vi "sql-readinfo_vfixture.vi"(0 "DBSet":T1={"Server"="172.20.23.107", "DB"="HTPSDB", "PSW"="data'songyy", "User"="sa"}, 5 "操作模式":T2(ring)=enum."查询数据", 7 "查询项目":string="LuxsharePN,CustomerPN,Customer,SampleDes,AWG,Length,EEPROMWrite,LabelPrint,Remarks", 11 "标识列":string, 12 "限定条件":string="where LuxsharePN='L12345678'", 13 "Page":string, 15 "Desc":string) -> (14 "数据输出2":dbl[][](array[numeric]), 16 "错误类型":string, 17 "StringArray2":string[][](array[string])=[["L12345678\t\tIBM\t40G Ethernet QSFP+ Passive DAC Cable\t28\t3000\t0\t0\trefer to IBM Spec"]], 18 "列内对数":i32=1, 19 "返回记录数目":i32=1, 20 "ConvertToArray":string[][](array[string])=[["L12345678", "", "IBM", "40G Ethernet QSFP+ Passive DAC Cable", "28", "3000", "0", "0", "refer to IBM Spec"]], 21 "status":bool, 23 "ResultString":string="L12345678\t\tIBM\t40G Ethernet QSFP+ Passive DAC Cable\t28\t3000\t0\t0\trefer to IBM Spec\r", 24 "ConvertToClusterArray":cluster{"项":string, "值":string}[](array[cluster])=[{"项"="", "值"=""}, {"项"="L12345678", "值"="L12345678"}], 25 "DataPair":dbl[](array[numeric]), 27 "数据输出":dbl[][](array[numeric]))   [LabVIEW 2011]
panel:
  out "错误输出 2":errorcluster caption="错误输出"
  out "result string":string="select LuxsharePN,CustomerPN,Customer,SampleDes,AWG,Length,EEPROMWrite,LabelPrint,Remarks from project where LuxsharePN='L12345678'"
  out "替换数量":i32=9
  in  "二级分隔符":string
  in  "一级分隔符":string
  in  "表名":string="vproject"
  out "Result":bool=TRUE
  in  "InitArray1":string[][](array[string])
  in  "MoveToTail":i32=1
  in  "InitArray2":string[](array[string])
  out "错误输出":errorcluster
  in  "初始化簇数组":cluster{"项":string, "值":string}[](array[cluster])
  in  "簇元素":cluster{"项":string, "值":string}
  in  "input-db":string="HTPSDB"
  in  "input-psw":string="htps'songyy"
  in  "input-user":string="htpsuser"
  in  "input-IP":string="sql2012agl01.luxshare.com.cn"
  in  "ADODB._Recordset":refnum<k7>
  in  "ADODB._Connection":refnum<k7>
  # "列名 & 表名 查询结果"
  # "输       出"
  # "输       入"
  # "基本信息\n（）"
  # "状态灯，False表示操作成功，True表示操作失败"
  # "簇数组"
  # "限定条件，设定某个条件，输出满足该条件的数据"
  # "对数"
  # "错误类型"
  # "查询记录时才需要填写，page用于设置查询一次请求的记录数，Desc用于截断Desc条记录之前的记录"
  # "改变操作时需要修改的信息"
  # "操作模式：查询表名\n                  查询列名\n                  查询记录\n                  查询总记录\n                  查询数据"
  # "字符串"
  # "数组"
  # "查询表名时不需要输入\n\n查询列名和查询数据时要指定哪一张表"
  # "字符串数组"
  # "在查询表名和列名时不需要输入信息\n\n在查询数据时，如果要输入所有列，填入“*”，如果要查询指定的某一个列，输入该列的名称"
  # "ProjectName"
  # "EEPROMContent"
  # "LimitSpec"
  # "LabelContent"
  # "SwitchMatrix"
  # "error:\n-2147217843 登陆失败： 。\n-2147467259 要访问的数据库不存在\n-2146825267 没有数据    。\n-2146824584 对象关闭时，不允许操作\n-2147217865 表名不存在 。\n-2147467259 服务器连接失败 。"
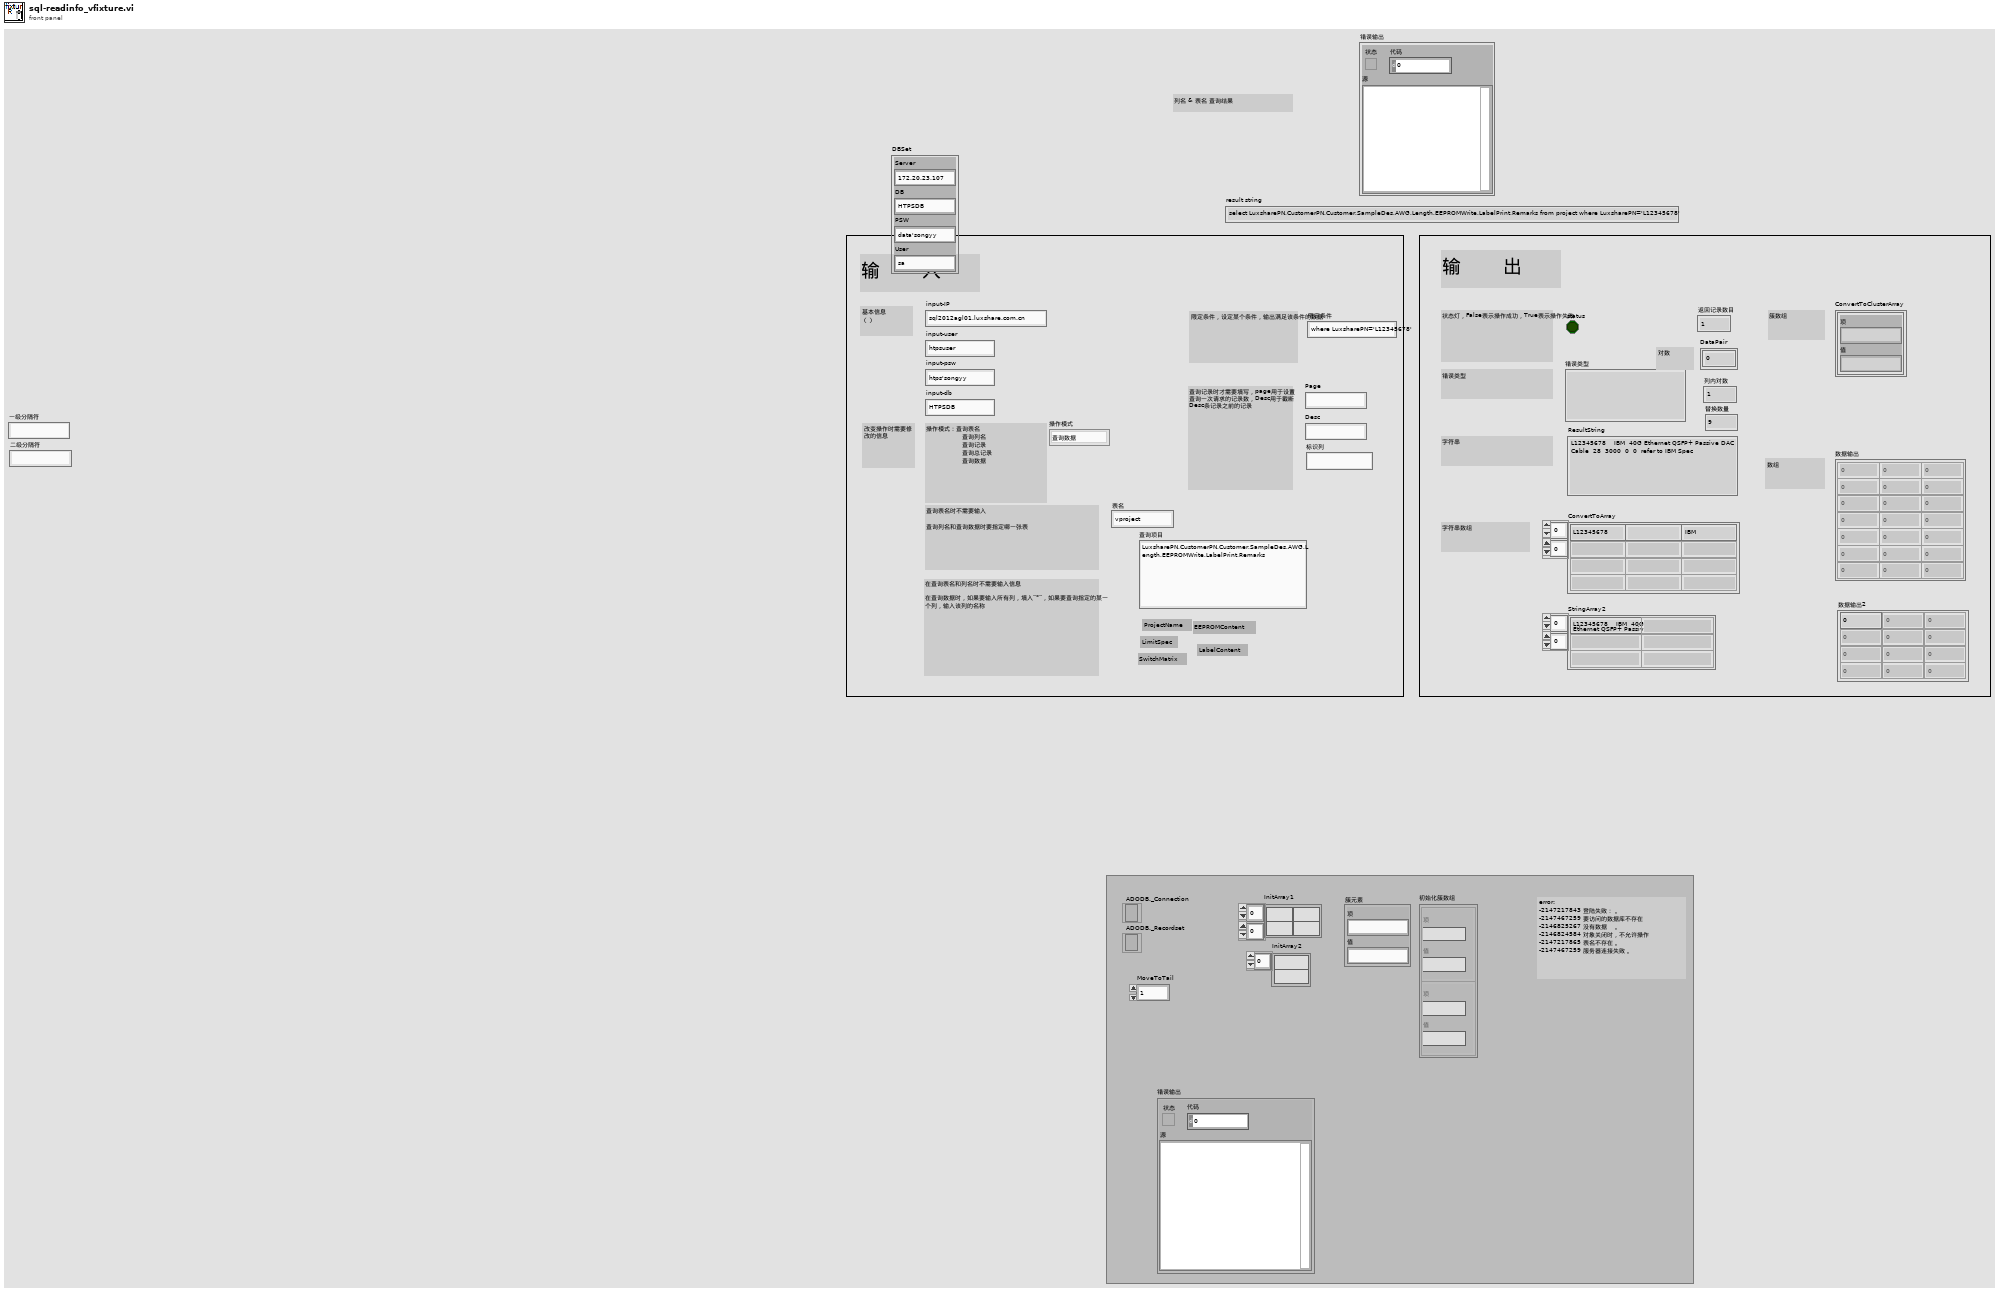
[diagram p1: front panel]
types:
  T1 = cluster{"Server":string, "DB":string, "PSW":string, "User":string}
  T2 = enum16{"查询表名", "查询列名", "查询记录", "查询总记录", "查询数据", "转换数据"}
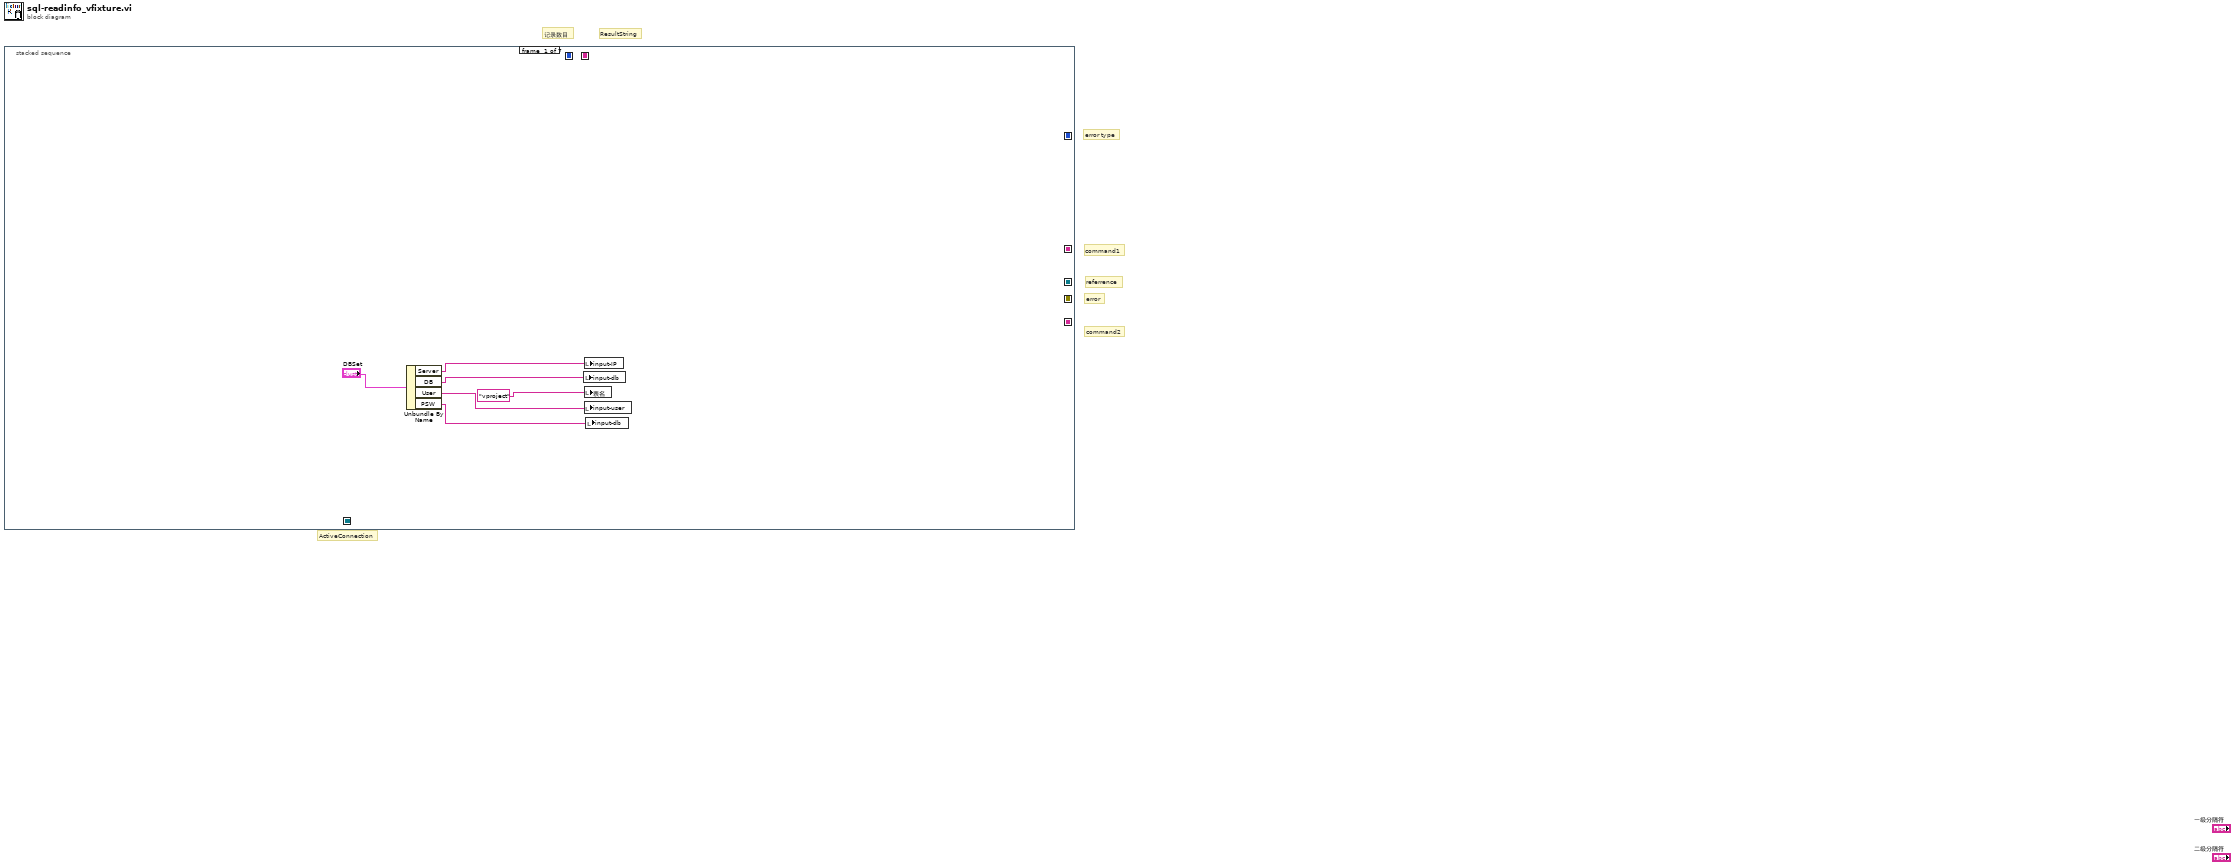
[diagram p0: block diagram]
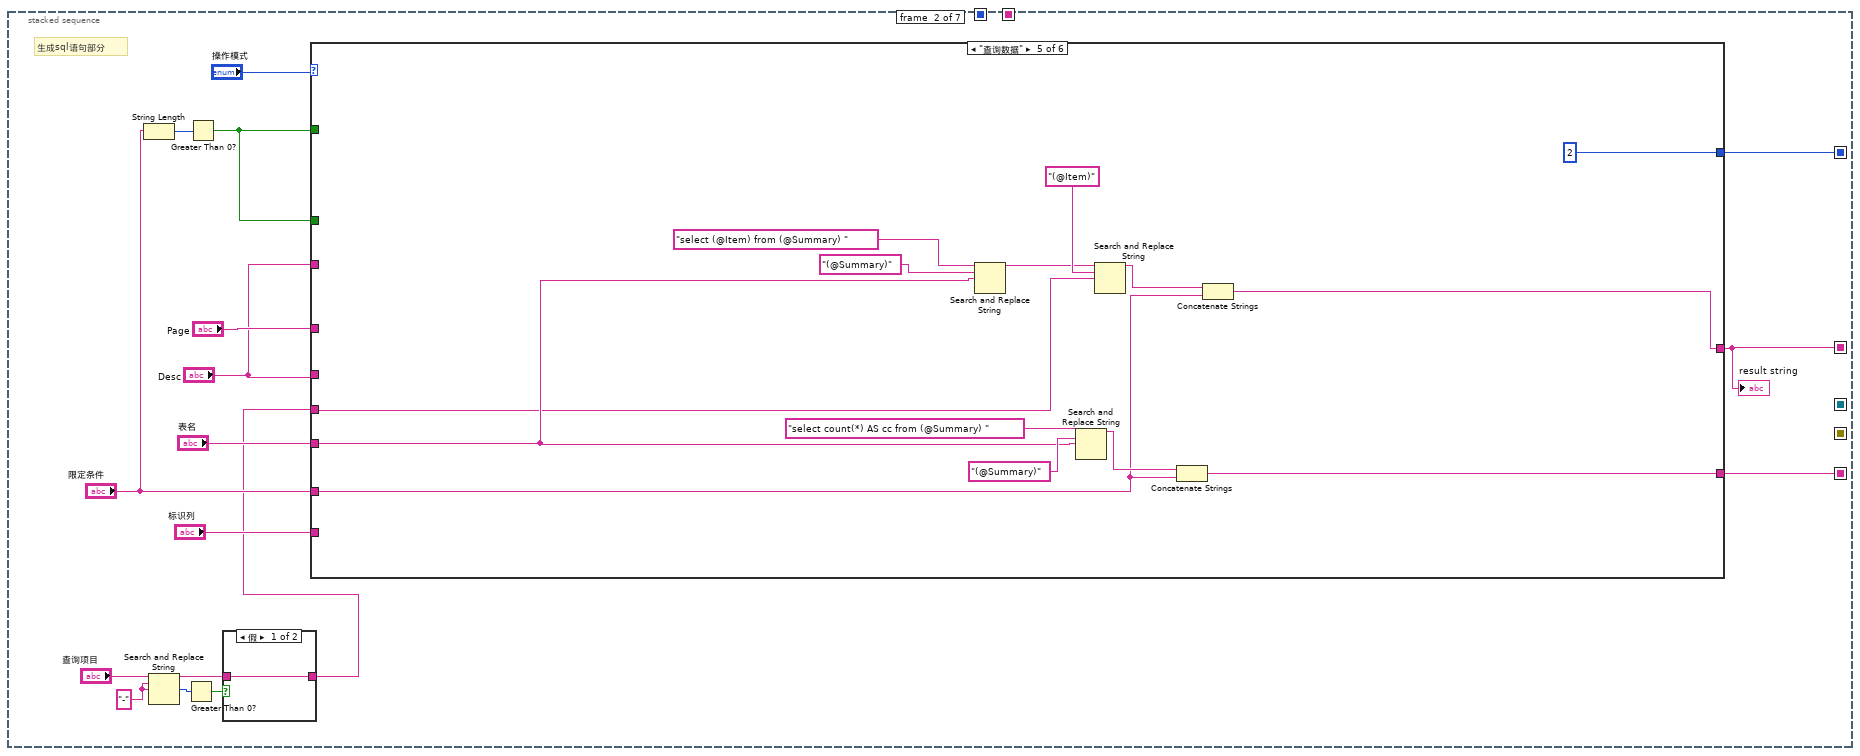
[diagram p2: hidden frame]
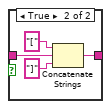
[diagram p3: hidden frame]
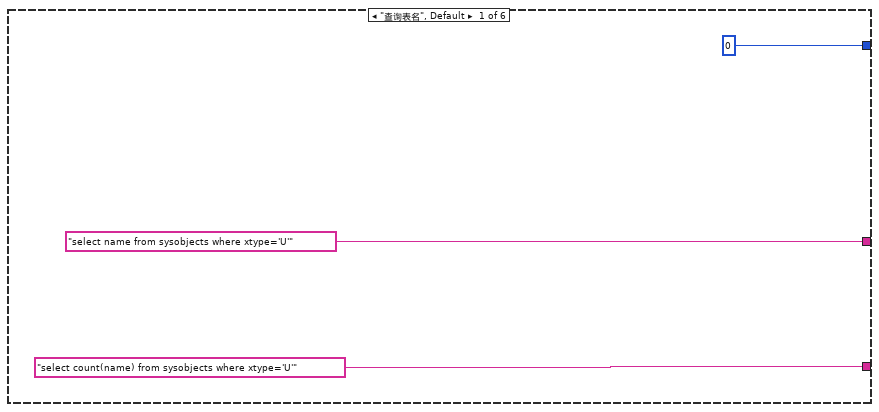
[diagram p4: hidden frame]
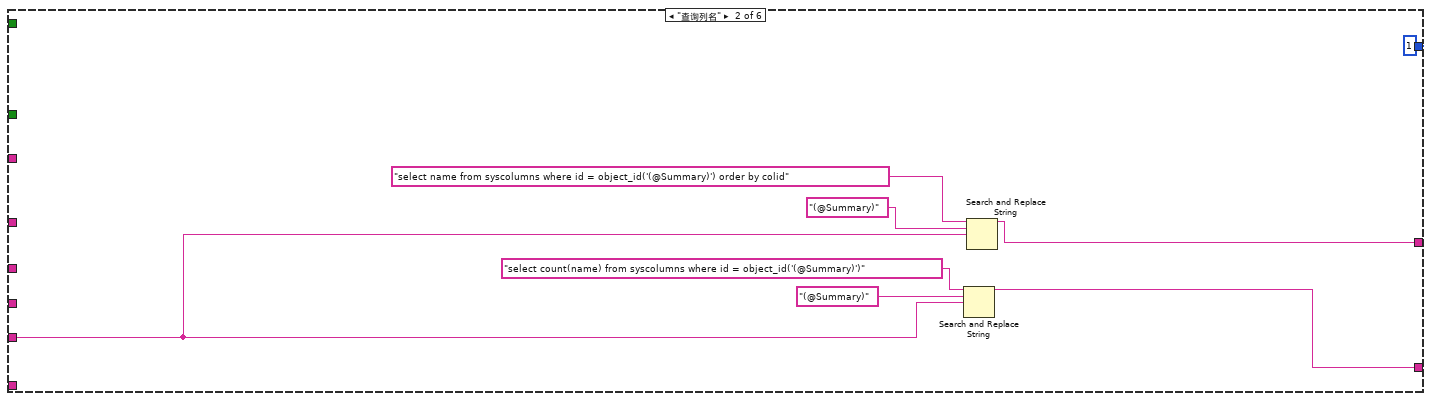
[diagram p5: hidden frame]
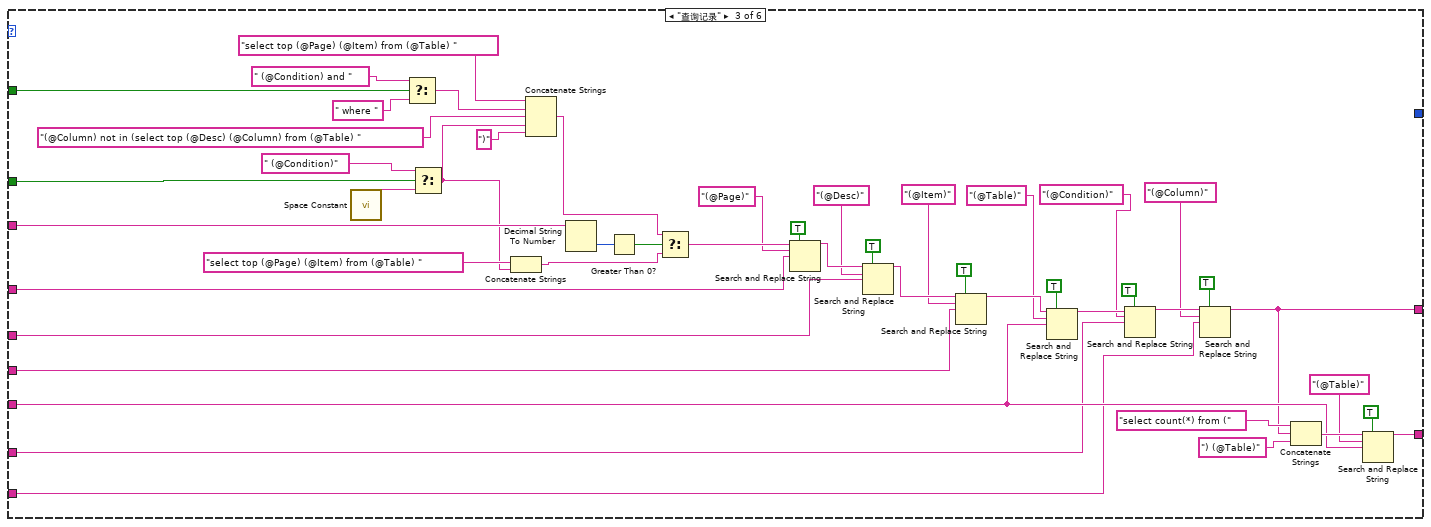
[diagram p6: hidden frame]
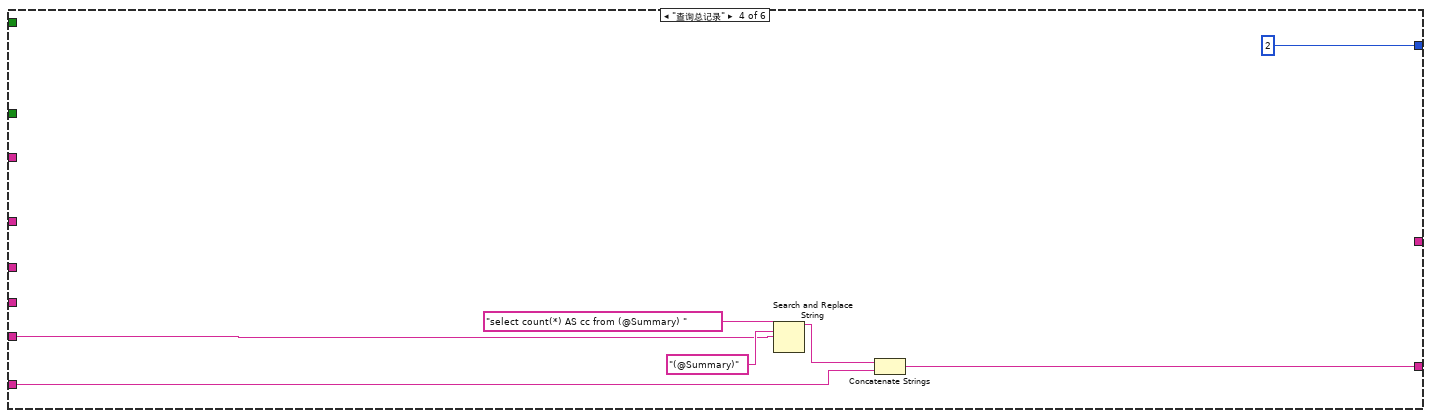
[diagram p7: hidden frame]
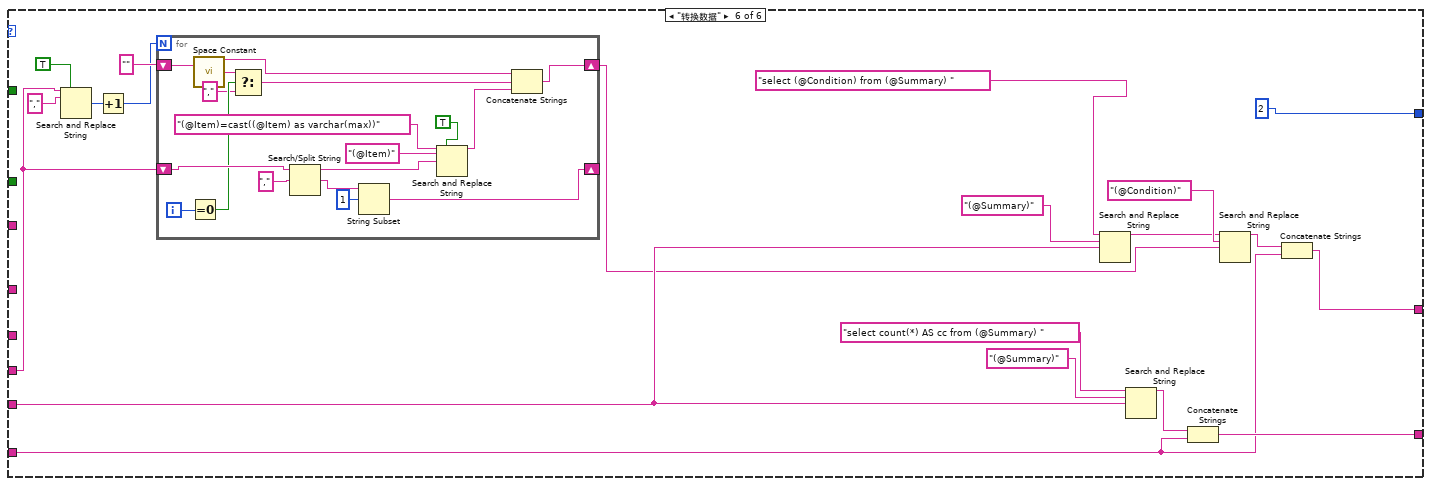
[diagram p8: hidden frame]
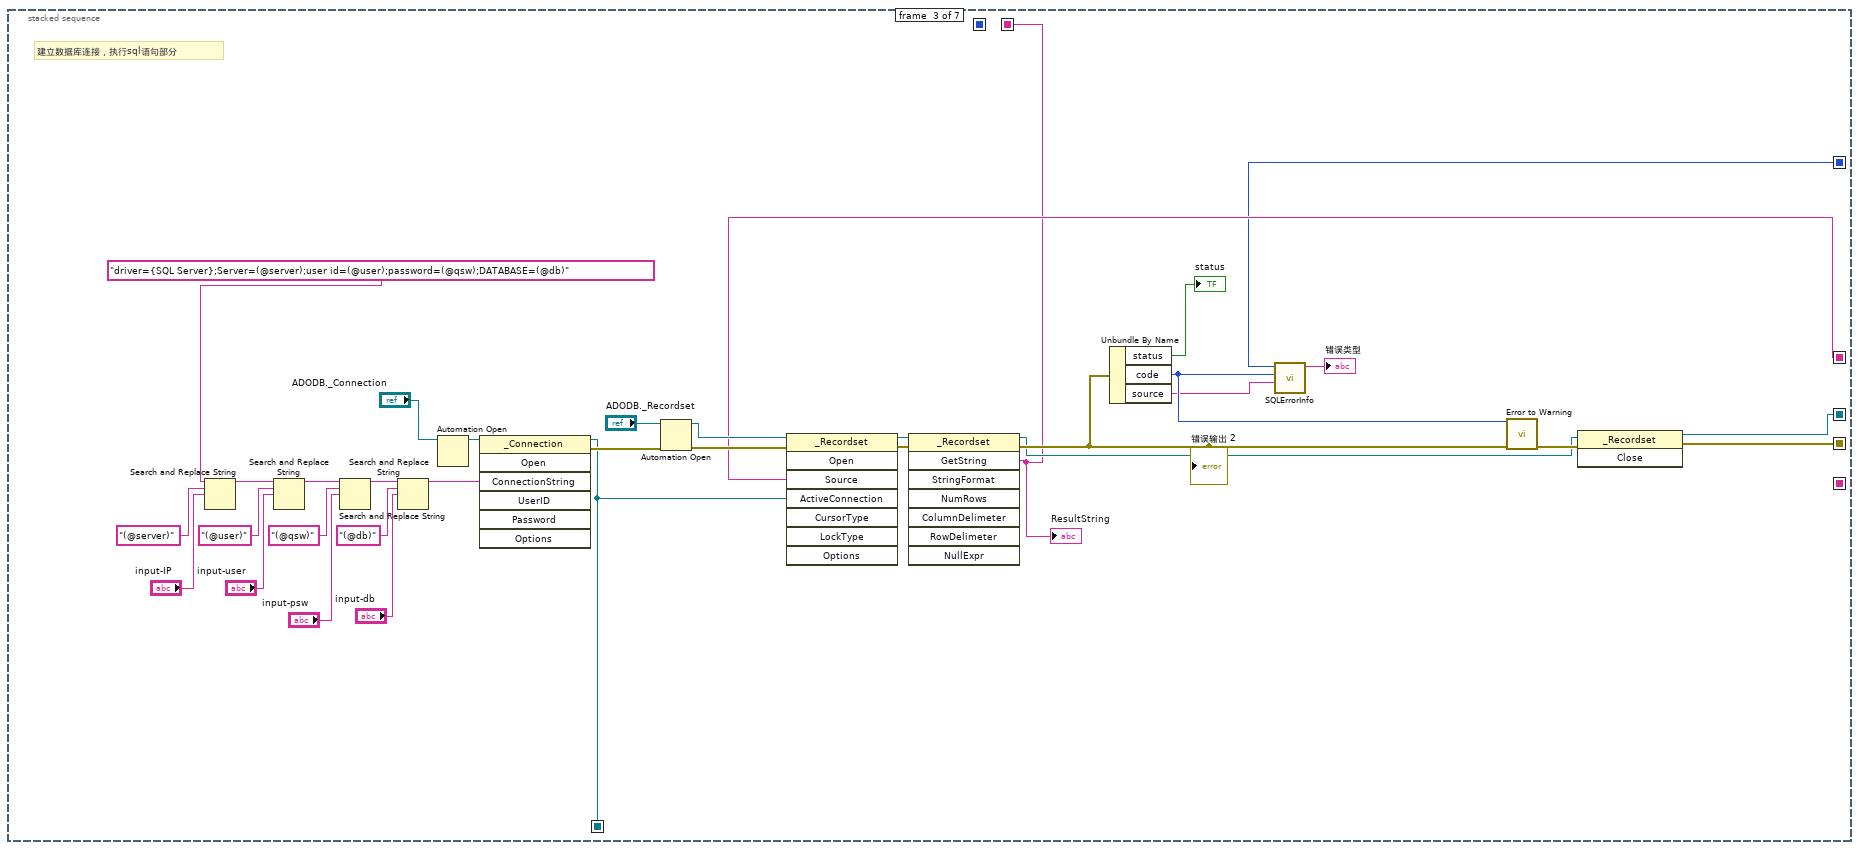
[diagram p9: hidden frame]
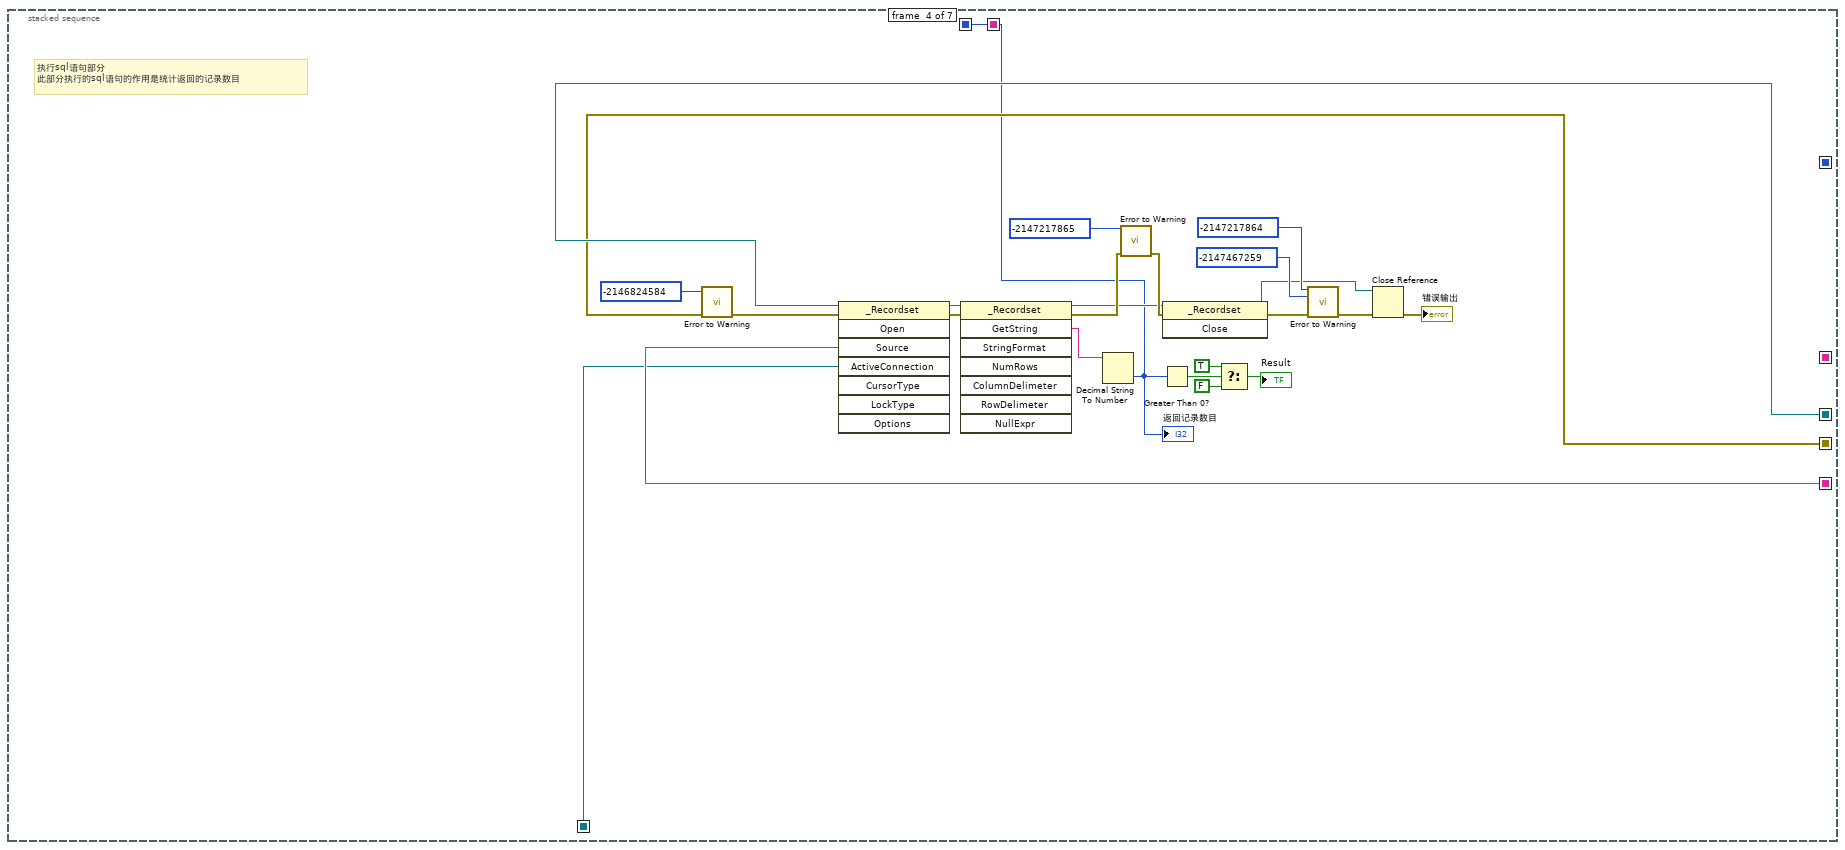
[diagram p10: hidden frame]
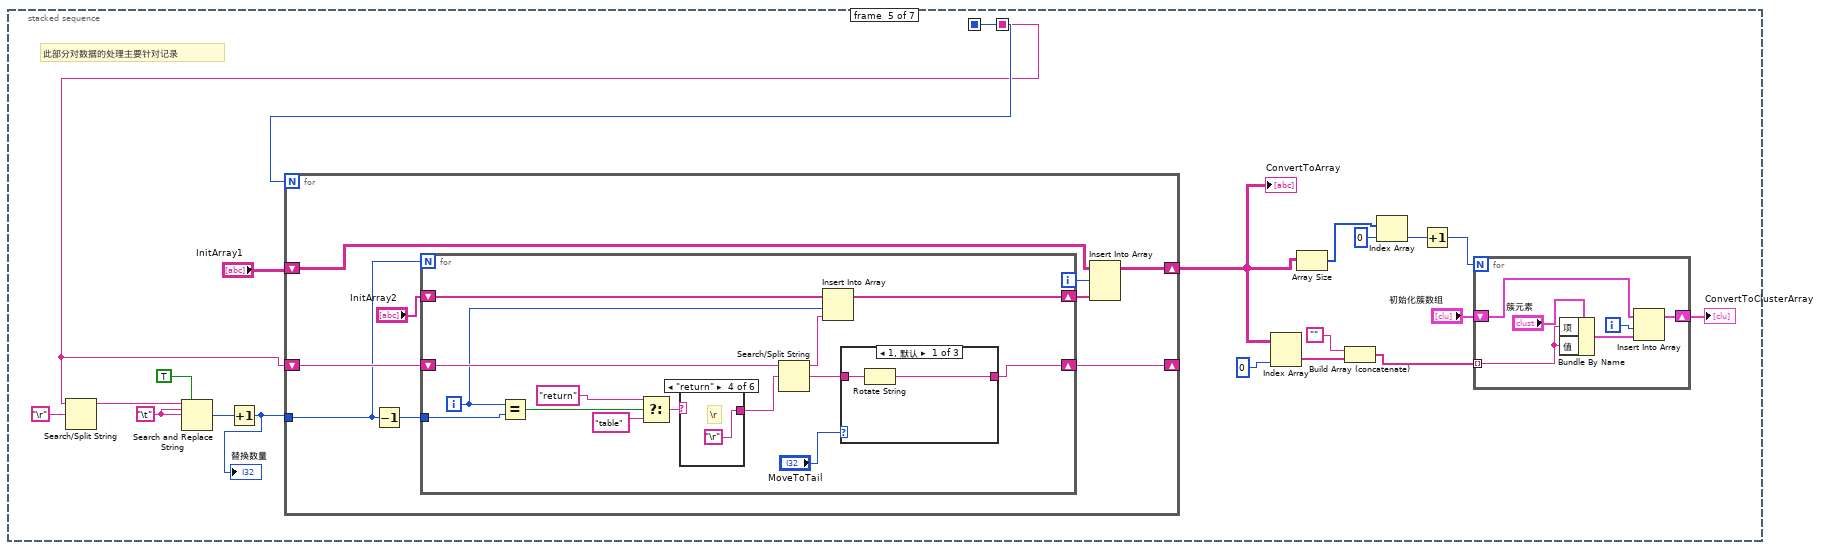
[diagram p11: hidden frame]
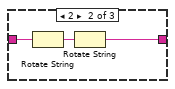
[diagram p12: hidden frame]
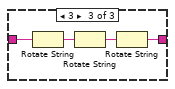
[diagram p13: hidden frame]
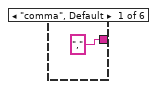
[diagram p14: hidden frame]
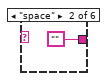
[diagram p15: hidden frame]
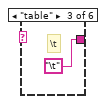
[diagram p16: hidden frame]
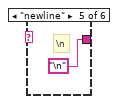
[diagram p17: hidden frame]
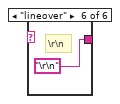
[diagram p18: hidden frame]
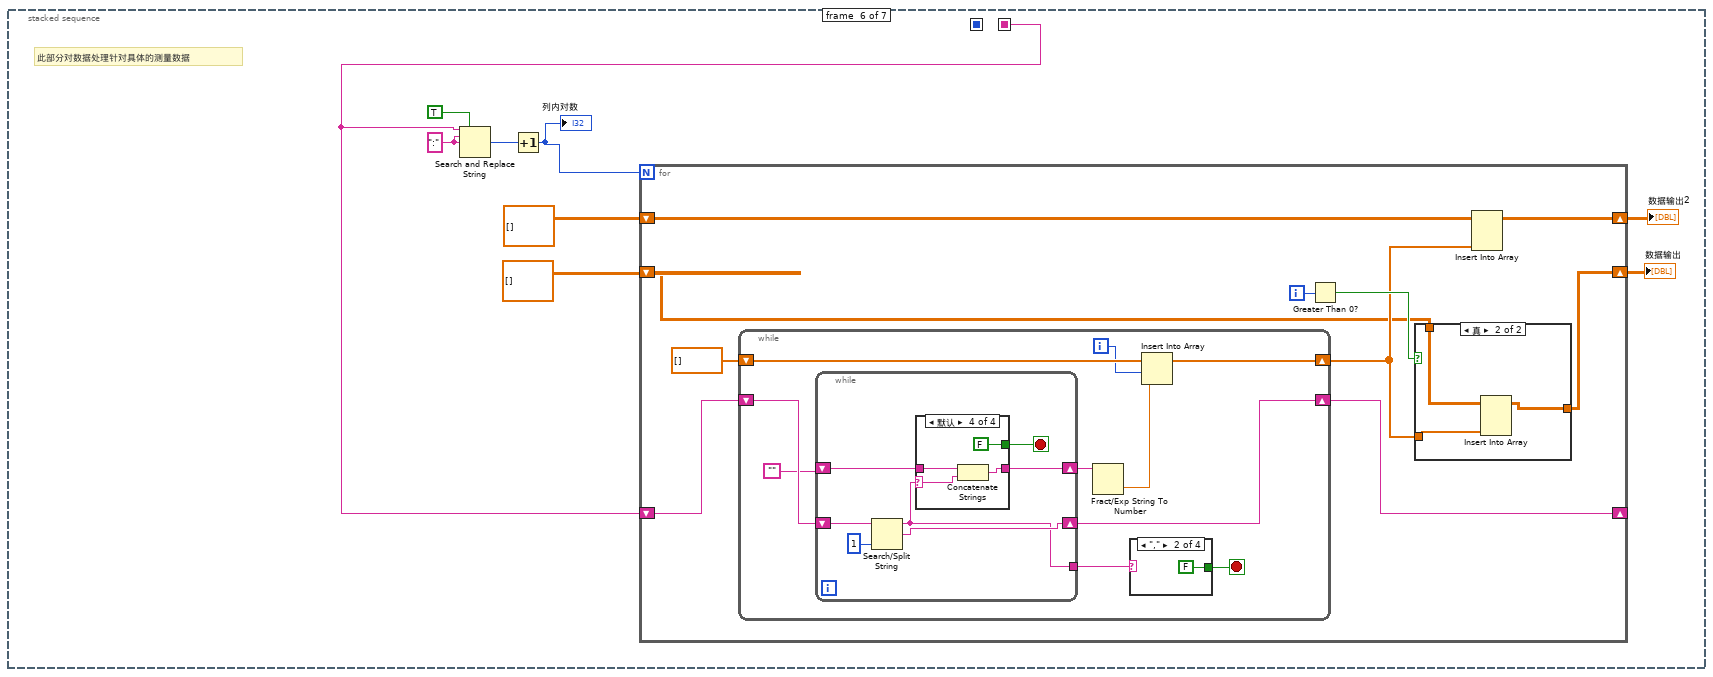
[diagram p19: hidden frame]
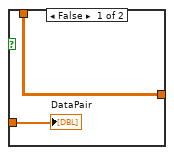
[diagram p20: hidden frame]
diagram:
  # "记录数目"
  # "ActiveConnection"
  # "referrence"
  # "error"
  # "error type"
  # "command2"
  # "command1"
  # "ResultString"
  n1 = stacked-sequence {
    seq-local: [_ _ w153 _ _ _ _] -> [_ _ _ w183 _ _ _]
    seq-local: [_ w11 _ _ _ _ _] -> [_ _ w149 _ _ _ _]
    seq-local: [_ w10 _ _ _ _ _] -> [_ _ w154 _ _ _ _]
    seq-local: [_ _ w152 _ _ _ _] -> [_ _ _ _ w204 w268 w324]
    seq-local: [_ _ w151 _ _ _ _] -> [_ _ _ w181 _ _ _]
    seq-local: [_ _ w150 _ _ _ _] -> [_ _ _ w182 _ _ _]
    seq-local: [_ w9 _ _ _ _ _] -> [_ _ _ w184 _ _ _]
    seq-local: [_ _ _ w180 _ _ _] -> [_ _ _ _ w205 _ _]
    frame #0 {
      n2 = Unbundle By Name("DBSet") -> ("Server"=w4:string, "DB"=w3:string, "User"=w1:string, "PSW"=w2:string)
      n3 = local write "input-db"(w3) -> ()
      n4 = local write "input-IP"(w4) -> ()
      n5 = local write "表名"("vproject") -> ()
      n6 = local write "input-user"(w1) -> ()
      n7 = local write "input-db"(w2) -> ()
    }
    frame #1 {
      w21 = "-"
      # "生成sql语句部分"
      n8 = String Length(string="限定条件") -> (length=w13:i32)
      n9 = Search and Replace String(input string="查询项目", search string=w21, replace string=w21) -> (result string=w18:string, number of replacements=w20:i32)  [unwired: 5 in, 2 out]
      n10 = Greater Than 0?(x=w20) -> (x > 0?=w19:bool)
      n11 = Greater Than 0?(x=w13) -> (x > 0?=w12:bool)
      n12 = case shown="假" w19 {
        tunnel: w18 -> [w24 w27]
        tunnel: [w24 w25] -> w7
        frame False {
        }
        frame True {
          n13 = Concatenate Strings("[", w27, "]") -> (w25:string)
        }
      }
      n14 = case shown="\"查询数据\"" "操作模式" {
        tunnel: "表名" -> [_ w36 w73 w92 w105 w117]
        tunnel: "限定条件" -> [_ _ w66 w89 w97 w120]
        tunnel: ["select name from sysobjects where xtype='U'" w34 w44 _ w98 w121] -> w10
        tunnel: ["select count(name) from sysobjects where xtype='U'" w35 w72 w90 w103 w125] -> w9
        tunnel: w7 -> [_ _ w78 _ w101 w110]
        tunnel: [0 1 _ 2 2 2] -> w11
        tunnel: "Page" -> [_ _ w85 _ _ _]
        tunnel: "Desc" -> [_ _ w84 _ _ _]
        tunnel: "Desc" -> [_ _ w64 _ _ _]
        tunnel: w12 -> [_ _ w60 _ _ _]
        tunnel: w12 -> [_ _ w56 _ _ _]
        tunnel: "标识列" -> [_ _ w40 _ _ _]
        frame "查询表名", Default {
        }
        frame "查询列名" {
          n15 = Search and Replace String(input string="select count(name) from syscolumns where id = object_id('(@Summary)')", search string="(@Summary)" ("搜索字符串"), replace string=w36) -> (result string=w35:string)  [unwired: 5 in, 3 out]
          n16 = Search and Replace String(input string="select name from syscolumns where id = object_id('(@Summary)') order by colid", search string="(@Summary)" ("搜索字符串"), replace string=w36) -> (result string=w34:string)  [unwired: 5 in, 3 out]
        }
        frame "查询记录" {
          n17 = call <vilib>:"Space Constant.vi"() -> ("String"=w57:string)
          n18 = Select(t=" (@Condition) and ", s=w60, f=" where ") -> (s? t:f=w54:string)
          n19 = Select(t=" (@Condition)", s=w56, f=w57) -> (s? t:f=w49:string)
          n20 = Concatenate Strings("select top (@Page) (@Item) from (@Table) ", w49) -> (w48:string)
          n21 = Concatenate Strings("select top (@Page) (@Item) from (@Table) ", w54, "(@Column) not in (select top (@Desc) (@Column) from (@Table) ", w49, ")") -> (w51:string)
          n22 = Decimal String To Number(string=w64) -> (number=w63:i32)  [unwired: 2 in, 1 out]
          n23 = Greater Than 0?(x=w63) -> (x > 0?=w62:bool)
          n24 = Select(t=w51, s=w62, f=w48) -> (s? t:f=w61:string)
          n25 = Search and Replace String(replace all?=TRUE ("替换全部？(F)"), input string=w61, search string="(@Page)" ("搜索字符串"), replace string=w85) -> (result string=w87:string)  [unwired: 4 in, 3 out]
          n26 = Search and Replace String(replace all?=TRUE ("替换全部？(F)"), input string=w87, search string="(@Desc)" ("搜索字符串"), replace string=w84) -> (result string=w81:string)  [unwired: 4 in, 3 out]
          n27 = Search and Replace String(replace all?=TRUE ("替换全部？(F)"), input string=w81, search string="(@Item)" ("搜索字符串"), replace string=w78) -> (result string=w76:string)  [unwired: 4 in, 3 out]
          n28 = Search and Replace String(replace all?=TRUE ("替换全部？(F)"), input string=w76, search string="(@Table)" ("搜索字符串"), replace string=w73) -> (result string=w68:string)  [unwired: 4 in, 3 out]
          n29 = Search and Replace String(replace all?=TRUE ("替换全部？(F)"), input string=w68, search string="(@Condition)" ("搜索字符串"), replace string=w66) -> (result string=w43:string)  [unwired: 4 in, 3 out]
          n30 = Search and Replace String(replace all?=TRUE ("替换全部？(F)"), input string=w43, search string="(@Column)" ("搜索字符串"), replace string=w40) -> (result string=w44:string)  [unwired: 4 in, 3 out]
          n31 = Concatenate Strings("select count(*) from (", w44, ") (@Table)") -> (w75:string)
          n32 = Search and Replace String(replace all?=TRUE ("替换全部？(F)"), input string=w75, search string="(@Table)" ("搜索字符串"), replace string=w73) -> (result string=w72:string)  [unwired: 4 in, 3 out]
        }
        frame "查询总记录" {
          n33 = Search and Replace String(input string="select count(*) AS cc from (@Summary) ", search string="(@Summary)" ("搜索字符串"), replace string=w92) -> (result string=w91:string)  [unwired: 5 in, 3 out]
          n34 = Concatenate Strings(w91, w89) -> (w90:string)
        }
        frame "查询数据" {
          n35 = Search and Replace String(input string="select (@Item) from (@Summary) ", search string="(@Summary)" ("搜索字符串"), replace string=w105) -> (result string=w99:string)  [unwired: 5 in, 3 out]
          n36 = Search and Replace String(input string="select count(*) AS cc from (@Summary) ", search string="(@Summary)" ("搜索字符串"), replace string=w105) -> (result string=w104:string)  [unwired: 5 in, 3 out]
          n37 = Search and Replace String(input string=w99, search string="(@Item)" ("搜索字符串"), replace string=w101) -> (result string=w100:string)  [unwired: 5 in, 3 out]
          n38 = Concatenate Strings(w104, w97) -> (w103:string)
          n39 = Concatenate Strings(w100, w97) -> (w98:string)
        }
        frame "转换数据" {
          n40 = Search and Replace String(replace all?=TRUE ("替换全部？(F)"), input string=w110, search string="," ("搜索字符串")) -> (number of replacements=w113:i32)  [unwired: 5 in, 3 out]
          n41 = Increment(x=w113) -> (x+1=w114:i32)
          n42 = for {
            N: w114 -> [_]
            shift-right: [w132] -> w111
            shift-left: "" -> [w133]
            shift-right: [w129] -> _
            shift-left: w110 -> [w144]
            i -> [w139]
            n43 = Equal To 0?(x=w139) -> (x = 0?=w138:bool)
            n44 = call <vilib>:"Space Constant.vi"() -> ("String"=w137:string)
            n45 = Select(t=w137, s=w138, f=",") -> (s? t:f=w135:string)
            n46 = Search/Split String(string=w144, search string/char (-)="," ("搜索字符串/字符(-)")) -> (substring before match=w141:string, match + rest of string=w131:string)  [unwired: 1 in, 1 out]
            n47 = String Subset(string=w131, offset (0)=1 ("偏移量(0)")) -> (substring=w129:string)  [unwired: 1 in]
            n48 = Search and Replace String(replace all?=TRUE ("替换全部？(F)"), input string="(@Item)=cast((@Item) as varchar(max))", search string="(@Item)", replace string=w141) -> (result string=w134:string)  [unwired: 4 in, 3 out]
            n49 = Concatenate Strings(w133, w135, w134) -> (w132:string)
          }
          n50 = Search and Replace String(input string="select (@Condition) from (@Summary) ", search string="(@Summary)" ("搜索字符串"), replace string=w117) -> (result string=w122:string)  [unwired: 5 in, 3 out]
          n51 = Search and Replace String(input string="select count(*) AS cc from (@Summary) ", search string="(@Summary)" ("搜索字符串"), replace string=w117) -> (result string=w126:string)  [unwired: 5 in, 3 out]
          n52 = Concatenate Strings(w126, w120) -> (w125:string)
          n53 = Search and Replace String(input string=w122, search string="(@Condition)" ("搜索字符串"), replace string=w111) -> (result string=w123:string)  [unwired: 5 in, 3 out]
          n54 = Concatenate Strings(w123, w120) -> (w121:string)
        }
      }
      "result string" <- w10
    }
    frame #2 {
      # "建立数据库连接，执行sql语句部分"
      n55 = Search and Replace String(input string="driver={SQL Server};Server=(@server);user id=(@user);password=(@qsw);DATABASE=(@db)" ("ConnectionString"), search string="(@server)" ("搜索字符串"), replace string="input-IP") -> (result string=w159:string)  [unwired: 5 in, 3 out]
      n56 = Search and Replace String(input string=w159, search string="(@user)" ("搜索字符串"), replace string="input-user") -> (result string=w162:string)  [unwired: 5 in, 3 out]
      n57 = Search and Replace String(input string=w162, search string="(@qsw)" ("搜索字符串"), replace string="input-psw") -> (result string=w165:string)  [unwired: 5 in, 3 out]
      n58 = Search and Replace String(input string=w165, search string="(@db)" ("搜索字符串"), replace string="input-db") -> (result string=w169:string)  [unwired: 5 in, 3 out]
      n59 = Automation Open(Automation Refnum="ADODB._Connection") -> (Automation Refnum=w155:refnum<k7>)  [unwired: 3 in, 1 out]
      n60 = invoke class="_Connection" method="Open"(reference=w155, "ConnectionString"=w169) -> (reference out=w153:refnum<k7>, error out=w172:errorcluster)  [unwired: 5 in, 5 out]
      n61 = Automation Open(error in (no error)=w172, Automation Refnum="ADODB._Recordset") -> (Automation Refnum=w171:refnum<k7>, error out=w173:errorcluster)  [unwired: 2 in]
      n62 = invoke class="_Recordset" method="Open"(reference=w171, error in=w173, "Source"=w154, "ActiveConnection"=w153) -> (reference out=w174:refnum<k7>, error out=w175:errorcluster)  [unwired: 4 in, 6 out]
      n63 = invoke class="_Recordset" method="GetString"(reference=w174, error in=w175) -> (reference out=w176:refnum<k7>, error out=w179:errorcluster, "GetString"=w152:string)  [unwired: 6 in, 5 out]
      "ResultString" <- w152
      "错误输出 2" <- w179
      n64 = Unbundle By Name(w179) -> ("status"=→"status":bool, "code"=w148:i32, "source"=w147:string)
      n65 = call "SQLErrorInfo.vi"("input_error"=w147, "input_int_int"=w148, "input_int_ext"=w149) -> ("字符串"=→"错误类型":string)  [unwired: 8 in]
      n66 = call <vilib>:"Error to Warning.vi"("1st Error to Convert"=w148, "error in"=w179) -> ("warning out"=w177:errorcluster)  [unwired: 13 in]
      n67 = invoke class="_Recordset" method="Close"(reference=w176, error in=w177) -> (reference out=w150:refnum<k7>, error out=w151:errorcluster)  [unwired: 1 in, 1 out]
    }
    frame #3 {
      # "执行sql语句部分\n此部分执行的sql语句的作用是统计返回的记录数目"
      n68 = call <vilib>:"Error to Warning.vi"("1st Error to Convert"=-2146824584, "error in"=w181) -> ("warning out"=w194:errorcluster)  [unwired: 13 in]
      n69 = invoke class="_Recordset" method="Open"(reference=w182, error in=w194, "Source"=w184, "ActiveConnection"=w183) -> (reference out=w189:refnum<k7>, error out=w193:errorcluster)  [unwired: 4 in, 6 out]
      n70 = invoke class="_Recordset" method="GetString"(reference=w189, error in=w193) -> (reference out=w191:refnum<k7>, error out=w196:errorcluster, "GetString"=w190:string)  [unwired: 6 in, 5 out]
      n71 = Decimal String To Number(string=w190) -> (number=w180:i32)  [unwired: 2 in, 1 out]
      "返回记录数目" <- w180
      n72 = call <vilib>:"Error to Warning.vi"("1st Error to Convert"=-2147217865, "error in"=w196) -> ("warning out"=w197:errorcluster)  [unwired: 13 in]
      n73 = Greater Than 0?(x=w180) -> (x > 0?=w185:bool)
      n74 = invoke class="_Recordset" method="Close"(reference=w191, error in=w197) -> (reference out=w192:refnum<k7>, error out=w200:errorcluster)  [unwired: 1 in, 1 out]
      n75 = Select(t=TRUE, s=w185, f=FALSE) -> (s? t:f=→"Result":bool)
      n76 = call <vilib>:"Error to Warning.vi"("1st Error to Convert"=-2147217864, "2nd Error to Convert"=-2147467259, "error in"=w200) -> ("warning out"=w201:errorcluster)  [unwired: 12 in]
      n77 = Close Reference(reference=w192, error in (no error)=w201) -> (error out=→"错误输出":errorcluster)
    }
    frame #4 {
      w220 = "\t"
      # "此部分对数据的处理主要针对记录"
      n78 = Search/Split String(string=w204, search string/char (-)="\r") -> (substring before match=w219:string)  [unwired: 1 in, 2 out]
      n79 = Search and Replace String(replace all?=TRUE ("替换全部？(F)"), input string=w219, search string=w220, replace string=w220) -> (number of replacements=w222:i32)  [unwired: 4 in, 3 out]
      n80 = Increment(x=w222) -> (x+1=w223:i32)
      "替换数量" <- w223
      n81 = for {
        N: w205 -> [_]
        shift-right: [w229] -> w216
        shift-left: "InitArray1" -> [w230]
        shift-right: [w226] -> _
        shift-left: w204 -> [w232]
        tunnel: w223 -> [w225]
        i -> [w227]
        n82 = Decrement(x=w225) -> (x-1=w224:i32)
        n83 = for {
          N: w225 -> [_]
          shift-right: [w241] -> w226
          shift-left: w232 -> [w245]
          shift-right: [w242] -> w228
          shift-left: "InitArray2" -> [w244]
          tunnel: w224 -> [w233]
          i -> [w238]
          n84 = Equal?(x=w238, y=w233) -> (x = y?=w237:bool)
          n85 = Select(t="return", s=w237, f="table") -> (s? t:f=w234:string)
          n86 = case shown="\"return\"" w234 {
            tunnel: ["," "" "\t" "\r" "\n" "\r\n"] -> w246
            frame "comma", Default {
            }
            frame "space" {
            }
            frame "table" {
              # "\\t"
            }
            frame "return" {
              # "\\r"
            }
            frame "newline" {
              # "\\n"
            }
            frame "lineover" {
              # "\\r\\n"
            }
          }
          n87 = Search/Split String(string=w245, search string/char (-)=w246) -> (substring before match=w243:string, match + rest of string=w240:string)  [unwired: 1 in, 1 out]
          n88 = Insert Into Array(array=w244, index=w238, new element=w243) -> (w242:string[])
          n89 = case shown="1, 默认" "MoveToTail" {
            tunnel: [w247 w249 w253] -> w241
            tunnel: w240 -> [w248 w250 w252]
            frame 1, Default {
              n90 = Rotate String(1:w248) -> (0:w247:string)
            }
            frame 2 {
              n91 = Rotate String(1:w250) -> (0:w251:string)
              n92 = Rotate String(1:w251) -> (0:w249:string)
            }
            frame 3 {
              n93 = Rotate String(1:w252) -> (0:w255:string)
              n94 = Rotate String(1:w255) -> (0:w254:string)
              n95 = Rotate String(1:w254) -> (0:w253:string)
            }
          }
        }
        n96 = Insert Into Array(array=w230, index (row)=w227, new element=w228) -> (w229:string[][])  [unwired: 1 in]
      }
      "ConvertToArray" <- w216
      n97 = Index Array(array=w216, index (col)=0 ("禁用的索引 (列)")) -> (element=w213:string[])  [unwired: 1 in]
      n98 = Array Size(array=w216) -> (size(s)=w209:i32[])
      n99 = Build Array (concatenate)("", w213) -> (w214:string[])
      n100 = Index Array(array=w209, index=0 ("索引")) -> (element=w211:i32)
      n101 = Increment(x=w211) -> (x+1=w217:i32)
      n102 = for {
        N: w217 -> [_]
        tunnel: w214 -> [w267] mode=indexing
        shift-right: [w264] -> w207
        shift-left: "初始化簇数组" -> [w265]
        i -> [w266]
        n103 = Bundle By Name(cluster="簇元素", "项"=w267, "值"=w267) -> (w262:cluster{"项":string, "值":string})
        n104 = Insert Into Array(array=w265, index=w266, new element=w262) -> (w264:cluster{"项":string, "值":string}[])
      }
      "ConvertToClusterArray" <- w207
    }
    frame #5 {
      w269 = ":" ("搜索字符串")
      # "此部分对数据处理针对具体的测量数据"
      n105 = Search and Replace String(replace all?=TRUE ("替换全部？(F)"), input string=w268, search string=w269, replace string=w269) -> (number of replacements=w271:i32)  [unwired: 4 in, 3 out]
      n106 = Increment(x=w271) -> (x+1=w276:i32)
      "列内对数" <- w276
      n107 = for {
        N: w276 -> [_]
        shift-right: [w285] -> _
        shift-left: w268 -> [w286]
        shift-right: [w283] -> w273
        shift-left: dbl[][] [] -> [w279]
        shift-right: [w277] -> w275
        shift-left: dbl[][] [] -> [w278]
        i -> [w282]
        n108 = while {
          shift-right: [w298] -> w280
          shift-left: dbl[] [] -> [w299]
          shift-right: [w300] -> w285
          shift-left: w286 -> [w301]
          i -> [w297]
          stop <- w295 stop-if-true
          n109 = while {
            shift-right: [w310] -> w300
            shift-left: w301 -> [w312]
            shift-right: [w308] -> w293
            shift-left: "" -> [w309]
            tunnel: [w306] -> w296
            stop <- w307 stop-if-true
            n110 = Search/Split String(string=w312, offset (0)=1 ("偏移量(0)")) -> (substring before match=w306:string, match + rest of string=w310:string)  [unwired: 1 in, 1 out]
            n111 = case shown="默认" w306 {
              selector: w306 -> [_ _ _ w321]
              tunnel: w309 -> [w313 w315 w318 w322]
              tunnel: [w313 w315 w318 w320] -> w308
              tunnel: [TRUE TRUE TRUE FALSE] -> w307
              frame ":" {
              }
              frame "," {
              }
              frame "" {
              }
              frame Default {
                n112 = Concatenate Strings(w322, w321) -> (w320:string)
              }
            }
          }
          n113 = Fract/Exp String To Number(string=w293) -> (number=w292:dbl)  [unwired: 3 in, 1 out]
          n114 = case shown="\",\"" w296 {
            tunnel: [TRUE FALSE TRUE TRUE] -> w295
            frame ":" {
            }
            frame "," {
            }
            frame "" {
            }
            frame Default {
            }
          }
          n115 = Insert Into Array(array=w299, index=w297, new element=w292) -> (w298:dbl[])
        }
        n116 = Greater Than 0?(x=w282) -> (x > 0?=w281:bool)
        n117 = case shown="真" w281 {
          tunnel: [w288 w291] -> w283
          tunnel: w279 -> [w288 w290]
          tunnel: w280 -> [w287 w289]
          frame False {
            "DataPair" <- w287
          }
          frame True {
            n118 = Insert Into Array(array=w290, new element=w289) -> (w291:dbl[][])  [unwired: 2 in]
          }
        }
        n119 = Insert Into Array(array=w278, new element=w280) -> (w277:dbl[][])  [unwired: 2 in]
      }
      "数据输出" <- w273
      "数据输出2" <- w275
    }
    frame #6 {
      (unwired) 0.0
      w325 = ":" ("搜索字符串")
      # "此部分对数据处理针对具体的测量数据"
      n120 = Search and Replace String(replace all?=TRUE ("替换全部？(F)"), input string=w324, search string=w325, replace string=w325) -> (number of replacements=w327:i32)  [unwired: 4 in, 3 out]
      n121 = Increment(x=w327) -> (x+1=w329:i32)
      n122 = for {
        N: w329 -> [_]
        shift-right: [w335] -> _
        shift-left: w324 -> [w336]
        shift-right: [w330] -> w323
        shift-left: string[][] [] -> [w331]
        i -> [w333]
        n123 = Greater Than 0?(x=w333) -> ()  [unwired: 1 out]
        n124 = while {
          shift-right: [w343] -> w332
          shift-left: string[] [] -> [w344]
          shift-right: [w345] -> w335
          shift-left: w336 -> [w346]
          i -> [w342]
          stop <- w340 stop-if-true
          n125 = while {
            shift-right: [w355] -> w345
            shift-left: w346 -> [w357]
            shift-right: [w353] -> w338
            shift-left: "" -> [w354]
            tunnel: [w351] -> w341
            stop <- w352 stop-if-true
            n126 = Search/Split String(string=w357, offset (0)=1 ("偏移量(0)")) -> (substring before match=w351:string, match + rest of string=w355:string)  [unwired: 1 in, 1 out]
            n127 = case shown="\"\"" w351 {
              selector: w351 -> [_ _ _ w366]
              tunnel: w354 -> [w358 w360 w363 w367]
              tunnel: [w358 w360 w363 w365] -> w353
              tunnel: [TRUE TRUE TRUE FALSE] -> w352
              frame ":" {
              }
              frame "," {
              }
              frame "" {
              }
              frame Default {
                n128 = Concatenate Strings(w367, w366) -> (w365:string)
              }
            }
          }
          n129 = call <vilib>:"Trim Whitespace.vi"("string"=w338) -> ("trimmed string"=w337:string)  [unwired: 1 in]
          n130 = case shown="\",\"" w341 {
            tunnel: [TRUE FALSE TRUE TRUE] -> w340
            frame ":" {
            }
            frame "," {
            }
            frame "" {
            }
            frame Default {
            }
          }
          n131 = Insert Into Array(array=w344, index=w342, new element=w337) -> (w343:string[])
        }
        n132 = Insert Into Array(array=w331, new element=w332) -> (w330:string[][])  [unwired: 2 in]
      }
      "StringArray2" <- w323
    }
  }
